vi "GDCM_ConvertFileToJpeg.vi"() -> ()   [LabVIEW 2013, in "Medimatic.lvlib"]
uses:
  Medimatic.lvlib
  C:/Users/Simon/Dropbox/Medimatic/ProjectVerLV2011/DICOM/GDCM-2.2.1-Windows-x86/bin/gdcm-sharp.dll
  Dropbox/Medimatic/ProjectVerLV2011/DICOM/GDCM-2.2.1-Windows-x86/bin/gdcm-sharp.dll
panel:
  out "CanCode":bool
  out "Change":bool
  in  "error in (no error)":errorcluster
  out "error out":errorcluster
  in  "OutFile":string
  in  "filename_native":string
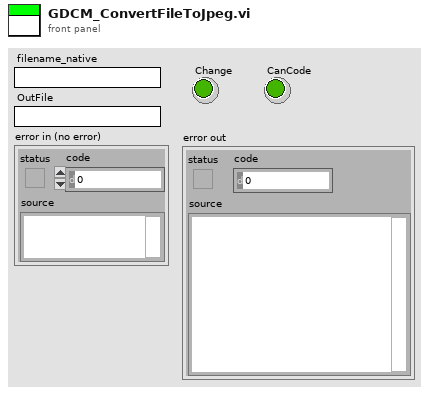
[diagram p1: front panel]
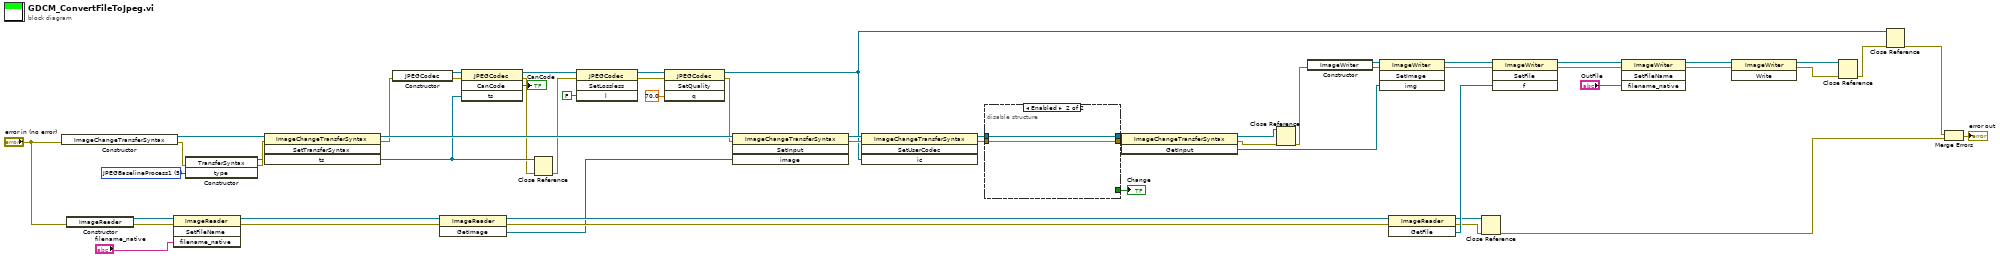
[diagram p0: block diagram]
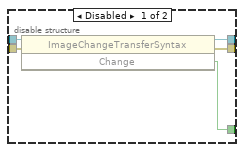
[diagram p2: hidden frame]
diagram:
  w53 = 5 items=["ImplicitVRLittleEndian", "ImplicitVRBigEndianPrivateGE", "ExplicitVRLittleEndian", "DeflatedExplicitVRLittleEndian", "ExplicitVRBigEndian", "JPEGBaselineProcess1", "JPEGExtendedProcess2_4", "JPEGExtendedProcess3_5", "JPEGSpectralSelectionProcess6_8", "JPEGFullProgressionProcess10_12", "JPEGLosslessProcess14", "JPEGLosslessProcess14_1", "JPEGLSLossless", "JPEGLSNearLossless", "JPEG2000Lossless", "JPEG2000", "RLELossless", "MPEG2MainProfile", "ImplicitVRBigEndianACRNEMA", "WeirdPapryus", "CT_private_ELE", "JPIPReferenced", "TS_END"] ("type")
  n1 = constructor class="ImageChangeTransferSyntax"(error in="error in (no error)") -> (reference out=w54:refnum<k24>, error out=w37:errorcluster)  [unwired: 2 in, 1 out]
  n2 = constructor class="ImageReader"(error in="error in (no error)") -> (reference out=w57:refnum<k24>, error out=w40:errorcluster)  [unwired: 2 in, 1 out]
  n3 = invoke class="ImageReader" method="SetFileName"(reference=w57, error in=w40, "filename_native"="filename_native") -> (reference out=w39:refnum<k24>, error out=w38:errorcluster)  [unwired: 1 in, 2 out]
  n4 = constructor class="TransferSyntax"(error in=w37, "type"=w53) -> (reference out=w16:refnum<k24>, error out=w36:errorcluster)  [unwired: 2 in, 2 out]
  n5 = invoke class="ImageChangeTransferSyntax" method="SetTransferSyntax"(reference=w54, error in=w36, "ts"=w16) -> (reference out=w48:refnum<k24>, error out=w33:errorcluster)  [unwired: 1 in, 2 out]
  n6 = constructor class="JPEGCodec"(error in=w33) -> (reference out=w55:refnum<k24>, error out=w35:errorcluster)  [unwired: 2 in, 1 out]
  n7 = invoke class="ImageReader" method="GetImage"(reference=w39, error in=w38) -> (reference out=w45:refnum<k24>, error out=w23:errorcluster, "GetImage"=w3:refnum<k24>)  [unwired: 1 in]
  n8 = invoke class="JPEGCodec" method="CanCode"(reference=w55, error in=w35, "ts"=w16) -> (reference out=w52:refnum<k24>, error out=w15:errorcluster, "CanCode"=→"CanCode":bool)  [unwired: 1 in, 1 out]
  n9 = Close Reference(reference=w16, error in (no error)=w15) -> (error out=w14:errorcluster)
  n10 = invoke class="JPEGCodec" method="SetLossless"(reference=w52, error in=w14, "l"=FALSE) -> (reference out=w50:refnum<k24>, error out=w34:errorcluster)  [unwired: 1 in, 2 out]
  n11 = invoke class="JPEGCodec" method="SetQuality"(reference=w50, error in=w34, "q"=70.0) -> (reference out=w13:refnum<k24>, error out=w32:errorcluster)  [unwired: 1 in, 2 out]
  n12 = invoke class="ImageChangeTransferSyntax" method="SetInput"(reference=w48, error in=w32, "image"=w3) -> (reference out=w47:refnum<k24>, error out=w29:errorcluster)  [unwired: 1 in, 2 out]
  n13 = invoke class="ImageChangeTransferSyntax" method="SetUserCodec"(reference=w47, error in=w29, "ic"=w13) -> (reference out=w31:refnum<k24>, error out=w28:errorcluster)  [unwired: 1 in, 2 out]
  n14 = disable-structure shown="Enabled" {
    disable-tunnel: w31 -> [w62 w64]
    disable-tunnel: [w61 w64] -> w30
    disable-tunnel: w28 -> [w60 w63]
    disable-tunnel: [w59 w63] -> w27
    disable-tunnel: [w58 _] -> w20
    frame Disabled {
      n15 = invoke class="ImageChangeTransferSyntax" method="Change"(reference=w62, error in=w60) -> (reference out=w61:refnum<k24>, error out=w59:errorcluster, "Change"=w58:bool)  [unwired: 1 in]
    }
    frame Enabled {
    }
  }
  "Change" <- w20
  n16 = invoke class="ImageChangeTransferSyntax" method="GetInput"(reference=w30, error in=w27) -> (reference out=w4:refnum<k24>, error out=w2:errorcluster, "GetInput"=w1:refnum<k24>)  [unwired: 1 in]
  n17 = Close Reference(reference=w4, error in (no error)=w2) -> (error out=w6:errorcluster)
  n18 = constructor class="ImageWriter"(error in=w6) -> (reference out=w46:refnum<k24>, error out=w26:errorcluster)  [unwired: 2 in, 1 out]
  n19 = invoke class="ImageWriter" method="SetImage"(reference=w46, error in=w26, "img"=w1) -> (reference out=w44:refnum<k24>, error out=w25:errorcluster)  [unwired: 1 in, 2 out]
  n20 = invoke class="ImageReader" method="GetFile"(reference=w45, error in=w23) -> (reference out=w10:refnum<k24>, error out=w9:errorcluster, "GetFile"=w43:refnum<k24>)  [unwired: 1 in]
  n21 = Close Reference(reference=w10, error in (no error)=w9) -> (error out=w8:errorcluster)
  n22 = invoke class="ImageWriter" method="SetFile"(reference=w44, error in=w25, "f"=w43) -> (reference out=w42:refnum<k24>, error out=w24:errorcluster)  [unwired: 1 in, 2 out]
  n23 = invoke class="ImageWriter" method="SetFileName"(reference=w42, error in=w24, "filename_native"="OutFile") -> (reference out=w19:refnum<k24>, error out=w18:errorcluster)  [unwired: 1 in, 2 out]
  n24 = invoke class="ImageWriter" method="Write"(reference=w19, error in=w18) -> (reference out=w17:refnum<k24>, error out=w11:errorcluster)  [unwired: 1 in, 1 out]
  n25 = Close Reference(reference=w17, error in (no error)=w11) -> (error out=w12:errorcluster)
  n26 = Close Reference(reference=w13, error in (no error)=w12) -> (error out=w7:errorcluster)
  n27 = Merge Errors(w7, w8) -> (→"error out":errorcluster)
